vi "Benchmark Convert String Type - Sizeof Strings.vi"(11 "conversions":T1[](array[typedef]) {"converted descriptor"."buffer offset" format="%d bytes"; "unconverted descriptor"."buffer offset" format="%d bytes"}) -> (2 "converted string size":u64, 3 "unconverted string size":u64)   [LabVIEW 2017]
uses:
  Classes/Buffer Converter/Type Conversion.ctl
  Classes/Buffer Converter/Channel Descriptor.ctl
  Typedefs/DSF Data Type.ctl
  VIs/Sizeof.vi
  DSF Core.lvlib
  Classes/Buffer/Buffer.lvclass
  Classes/Buffer Converter/Buffer Converter.lvclass
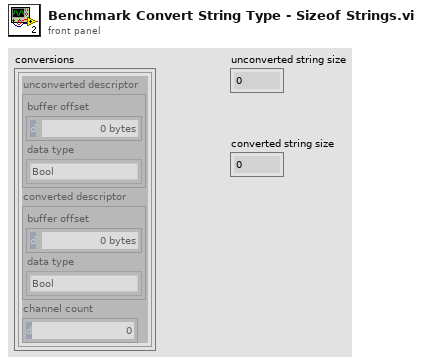
[diagram p1: front panel]
types:
  T1 = typedef "DSF Core.lvlib/Buffer Converter.lvclass/Type Conversion.ctl" = cluster{"unconverted descriptor":T2, "converted descriptor":T2, "channel count":u64}
  T2 = typedef "DSF Core.lvlib/Buffer.lvclass/Channel Descriptor.ctl" = cluster{"buffer offset":u64, "data type":T3}
  T3 = typedef "DSF Core.lvlib/DSF Data Type.ctl" = enum8{"Bool", "SGL", "DBL", "I8", "I16", "I32", "I64", "U8", "U16", "U32", "U64"}
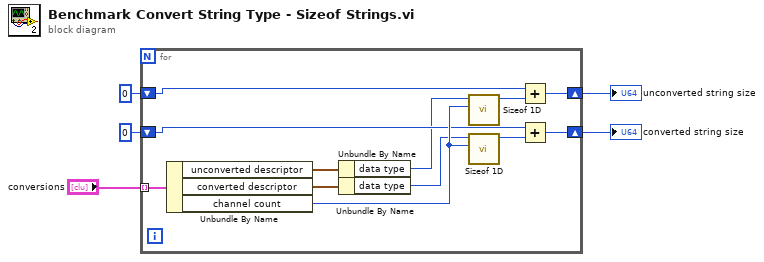
[diagram p0: block diagram]
diagram:
  n1 = for {
    tunnel: "conversions" -> [w17] mode=indexing
    shift-right: [w9] -> w1
    shift-left: u64 0 ("size in bytes") -> [w8]
    shift-right: [w13] -> w2
    shift-left: u64 0 ("size in bytes") -> [w11]
    n2 = Unbundle By Name(w17) -> ("unconverted descriptor"=w16:T2, "converted descriptor"=w15:T2, "channel count"=w14:u64)
    n3 = Unbundle By Name(w16) -> ("data type"=w6:T3)
    n4 = Unbundle By Name(w15) -> ("data type"=w7:T3)
    n5 = call "Sizeof 1D.vi"("count"=w14, "data type"=w6) -> ("size in bytes"=w12:u64)  [unwired: 9 in]
    n6 = call "Sizeof 1D.vi"("count"=w14, "data type"=w7) -> ("size in bytes"=w10:u64)  [unwired: 9 in]
    n7 = Add(x=w11, y=w12) -> (x+y=w13:u64)
    n8 = Add(x=w8, y=w10) -> (x+y=w9:u64)
  }
  "unconverted string size" <- w2
  "converted string size" <- w1
